vi "Broadcast Refnum.vi"(8 "error in":errorcluster) -> (0 "error out":errorcluster, 3 "Broadcast Refnum":T1)   [LabVIEW 2020, in "SECS Scenarios.lvlib" / "Scenarios Class.lvclass"]
uses:
  Scenarios Class.lvclass
  Broadcast Refnum.ctl
  13-EnableDisable Alarm.ctl
  15-Process Program Request.ctl
  16-Process Program Send.ctl
  SECS Communication/S7 Message Class/S7F4.ctl
  17-Deleting a Process Program by Host.ctl
  SECS Communication/S7 Message Class/S7F18.ctl
  18-Host Requests Equipment Process Program Directory.ctl
  19-Equipment Process Program Uploading.ctl
  SECS Communication/SECS-II Class/Format Code.ctl
  20[1]-Process Program Downloading.ctl
  SECS Communication/S7 Message Class/S7F2.ctl
  20[2]-Process Program Downloading.ctl
  SECS Communication/S7 Message Class/S7F23.ctl
  SECS Communication/S7 Message Class/S7F24.ctl
  22-Host Sends Information to Equipment.ctl
  SECS Communication/S10 Message Class/S10F4.ctl
  26-Host Requests to Enter OFF-Line.ctl
  27-Host Requests to Enter On-Line.ctl
  SECS Communication/S1 Message Class/S1F18.ctl
  28[1]-Remote Control[PP-SELECT].ctl
  28[2]-Remote Control[START].ctl
  28[3]-Remote Control[STOP].ctl
  28[4]-Remote Control[LOCAL].ctl
  28[5]-Remote Control[REMOTE].ctl
  28[6]-Remote Control[RCMD].ctl
  SECS Communication/S2 Message Class/S2F41.ctl
  SECS Communication/S2 Message Class/S2F42.ctl
  30-Host Requests Equipment to Set Time.ctl
  SECS Communication/S2 Message Class/S2F32.ctl
  31-Host Requests Time Value from Equipment.ctl
  32[1]-Trace Data Collection.ctl
  32[2]-Trace Data Collection.ctl
  SECS Communication/S2 Message Class/S2F24.ctl
  SECS Communication/S7 Message Class/S7 Message Class.lvclass
  SECS Communication/SECS-II Class/SECS-II Class.lvclass
  SECS Communication/S10 Message Class/S10 Message Class.lvclass
  SECS Communication/S1 Message Class/S1 Message Class.lvclass
  <vilib>/Utility/Data Type/NI_Data Type.lvlib
  SECS Communication/S2 Message Class/S2 Message Class.lvclass
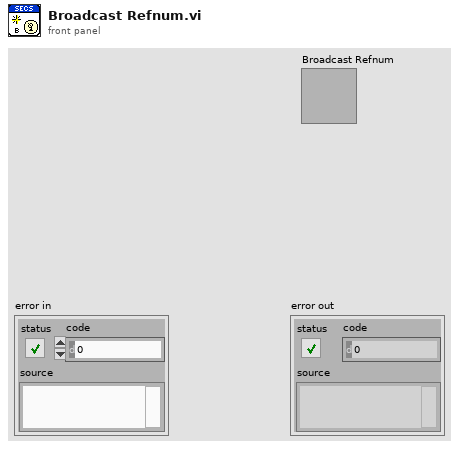
[diagram p1: front panel]
types:
  T1 = typedef "SECS Scenarios.lvlib/Scenarios Class.lvclass/Broadcast Refnum.ctl" = cluster{"13-EnableDisable Alarm":refnum<user-event>, "15-Process Program Request":refnum<user-event>, "16-Process Program Send":refnum<user-event>, "17-Deleting a Process Program by Host":refnum<user-event>, "18-Host Requests Equipment Process Program Directory":refnum<user-event>, "19-Equipment Process Program Uploading":refnum<user-event>, "20[1]-Process Program Downloading":refnum<user-event>, "20[2]-Process Program Downloading":refnum<user-event>, "22-Host Sends Information to Equipment":refnum<user-event>, "26-Host Requests to Enter OFF-Line":refnum<user-event>, "27-Host Requests to Enter On-Line":refnum<user-event>, "28[1]-Remote Control[PP-SELECT]":refnum<user-event>, "28[2]-Remote Control[START]":refnum<user-event>, "28[3]-Remote Control[STOP]":refnum<user-event>, "28[4]-Remote Control[LOCAL]":refnum<user-event>, "28[5]-Remote Control[REMOTE]":refnum<user-event>, "28[6]-Remote Control[RCMD]":refnum<user-event>, "30-Host Requests Equipment to Set Time":refnum<user-event>, "31-Host Requests Time Value from Equipment":refnum<user-event>, "32[1]-Trace Data Collection":refnum<user-event>, "32[2]-Trace Data Collection":refnum<user-event>}
  T2 = typedef "SECS Scenarios.lvlib/Scenarios Class.lvclass/13-EnableDisable Alarm.ctl" = cluster{"ALED":bool, "ALID":u32, "Reply Notifier":refnum<notifier>}
  T3 = typedef "SECS Scenarios.lvlib/Scenarios Class.lvclass/15-Process Program Request.ctl" = cluster{"PPID":string, "Reply Notifier":refnum<notifier>}
  T4 = typedef "SECS Scenarios.lvlib/Scenarios Class.lvclass/16-Process Program Send.ctl" = cluster{"PPID":string, "PPBODY":u8[], "Reply Notifier":refnum<notifier>}
  T5 = typedef "SECS Scenarios.lvlib/Scenarios Class.lvclass/17-Deleting a Process Program by Host.ctl" = cluster{"PPID":string[], "Reply Notifier":refnum<notifier>}
  T6 = typedef "SECS Scenarios.lvlib/Scenarios Class.lvclass/18-Host Requests Equipment Process Program Directory.ctl" = cluster{"Reply Notifier":refnum<notifier>}
  T7 = typedef "SECS Scenarios.lvlib/Scenarios Class.lvclass/19-Equipment Process Program Uploading.ctl" = cluster{"PPID":string, "Reply Notifier":refnum<notifier>}
  T8 = typedef "SECS Scenarios.lvlib/Scenarios Class.lvclass/20[1]-Process Program Downloading.ctl" = cluster{"PPID":string, "LENGTH":u32, "Reply Notifier":refnum<notifier>}
  T9 = typedef "SECS Scenarios.lvlib/Scenarios Class.lvclass/20[2]-Process Program Downloading.ctl" = cluster{"S7F23":T10, "Reply Notifier":refnum<notifier>}
  T10 = typedef "SECS Communication.lvlib/S7 Message Class.lvclass/S7F23.ctl" = cluster{"PPID":string, "MDLN":string, "SOFTREV":string, "Parameter":cluster{"CCODE":string, "PPARM":cluster{"Format Code":T11, "Value":variant}[]}[]}
  T11 = typedef "SECS Communication.lvlib/SECS-II Class.lvclass/Format Code.ctl" = enum16{"L", "A", "B", "Boolean", "J", "I1", "I2", "I4", "I8", "U1", "U2", "U4", "U8", "F4", "F8", "Char"}
  T12 = typedef "SECS Scenarios.lvlib/Scenarios Class.lvclass/22-Host Sends Information to Equipment.ctl" = cluster{"TID":u8, "TEXT":string, "Reply Notifier":refnum<notifier>}
  T13 = typedef "SECS Scenarios.lvlib/Scenarios Class.lvclass/26-Host Requests to Enter OFF-Line.ctl" = cluster{"Off-Line":bool, "Reply Notifier":refnum<notifier>}
  T14 = typedef "SECS Scenarios.lvlib/Scenarios Class.lvclass/27-Host Requests to Enter On-Line.ctl" = cluster{"On-Line":bool, "Reply Notifier":refnum<notifier>}
  T15 = typedef "SECS Scenarios.lvlib/Scenarios Class.lvclass/28[1]-Remote Control[PP-SELECT].ctl" = cluster{"PPID":string, "Reply Notifier":refnum<notifier>}
  T16 = typedef "SECS Scenarios.lvlib/Scenarios Class.lvclass/28[2]-Remote Control[START].ctl" = cluster{"Reply Notifier":refnum<notifier>}
  T17 = typedef "SECS Scenarios.lvlib/Scenarios Class.lvclass/28[3]-Remote Control[STOP].ctl" = cluster{"Reply Notifier":refnum<notifier>}
  T18 = typedef "SECS Scenarios.lvlib/Scenarios Class.lvclass/28[4]-Remote Control[LOCAL].ctl" = cluster{"Reply Notifier":refnum<notifier>}
  T19 = typedef "SECS Scenarios.lvlib/Scenarios Class.lvclass/28[5]-Remote Control[REMOTE].ctl" = cluster{"Reply Notifier":refnum<notifier>}
  T20 = typedef "SECS Scenarios.lvlib/Scenarios Class.lvclass/28[6]-Remote Control[RCMD].ctl" = cluster{"S2F41":T21, "Reply Notifier":refnum<notifier>}
  T21 = typedef "SECS Communication.lvlib/S2 Message Class.lvclass/S2F41.ctl" = cluster{"RCMD":string, "Parameter":cluster{"CPNAME":string, "CPVAL":string}[]}
  T22 = typedef "SECS Scenarios.lvlib/Scenarios Class.lvclass/30-Host Requests Equipment to Set Time.ctl" = cluster{"Time":string, "Reply Notifier":refnum<notifier>}
  T23 = typedef "SECS Scenarios.lvlib/Scenarios Class.lvclass/31-Host Requests Time Value from Equipment.ctl" = cluster{"Reply Notifier":refnum<notifier>}
  T24 = typedef "SECS Scenarios.lvlib/Scenarios Class.lvclass/32[1]-Trace Data Collection.ctl" = cluster{"Terminate TRID":u32}
  T25 = typedef "SECS Scenarios.lvlib/Scenarios Class.lvclass/32[2]-Trace Data Collection.ctl" = cluster{"TRID":u32, "DSPER":string, "TOTSMP":u32, "REPGSZ":u32, "SVID":u32[], "Reply Notifier":refnum<notifier>}
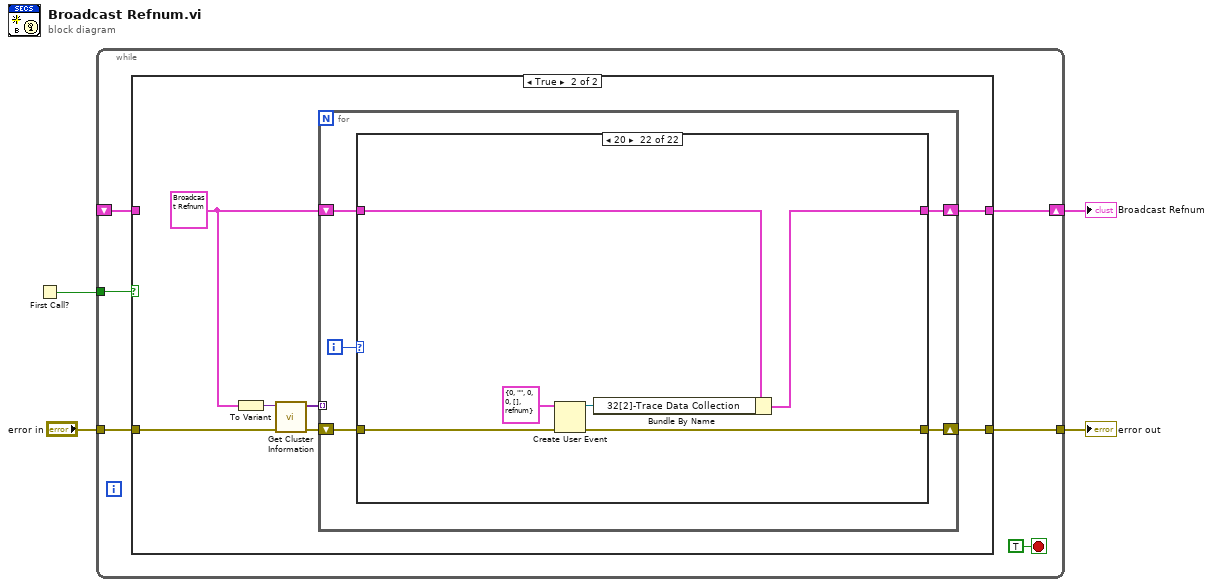
[diagram p0: block diagram]
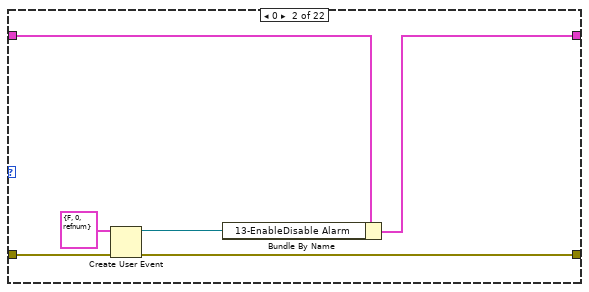
[diagram p4: hidden frame]
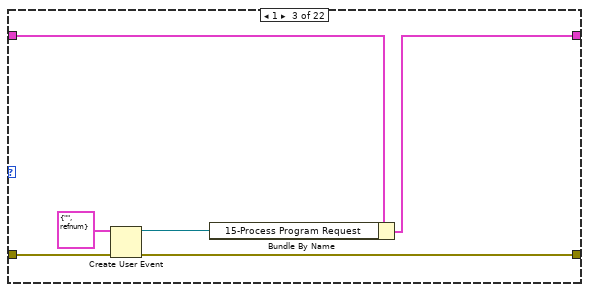
[diagram p5: hidden frame]
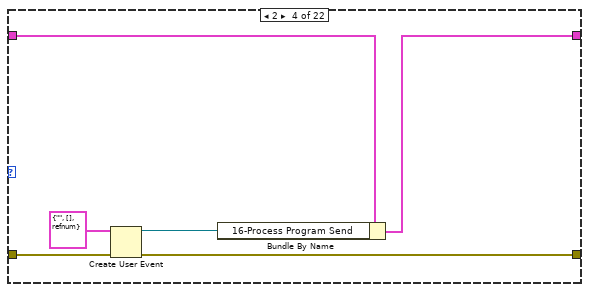
[diagram p6: hidden frame]
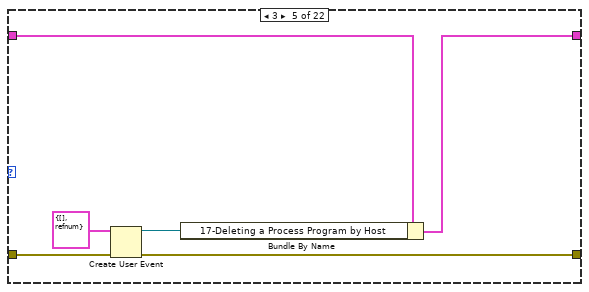
[diagram p7: hidden frame]
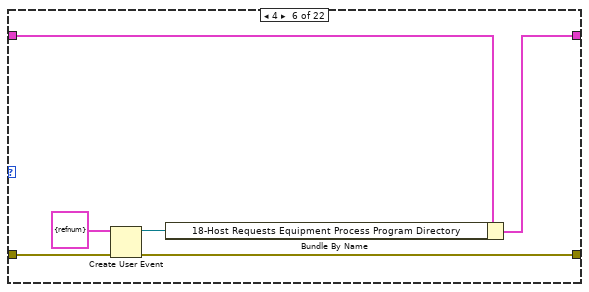
[diagram p8: hidden frame]
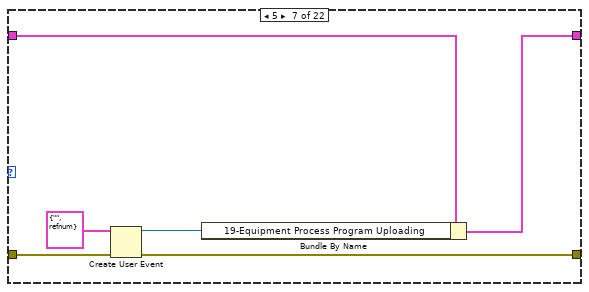
[diagram p9: hidden frame]
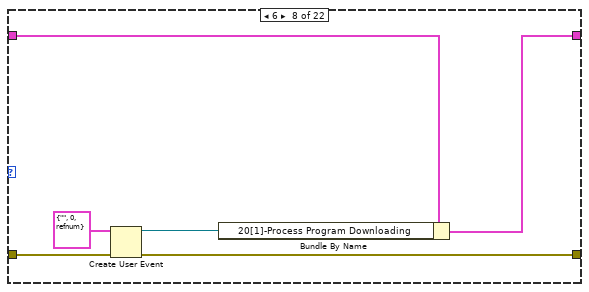
[diagram p10: hidden frame]
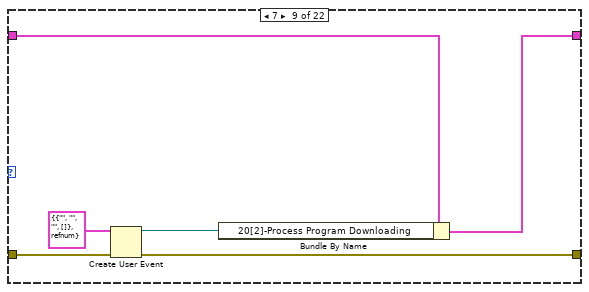
[diagram p11: hidden frame]
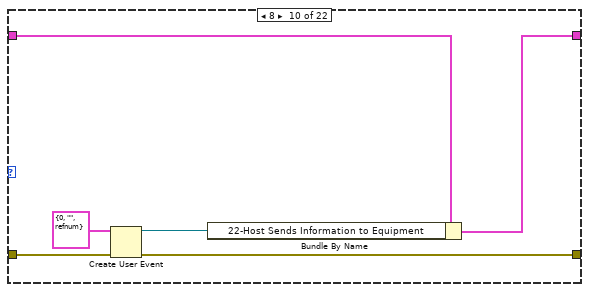
[diagram p12: hidden frame]
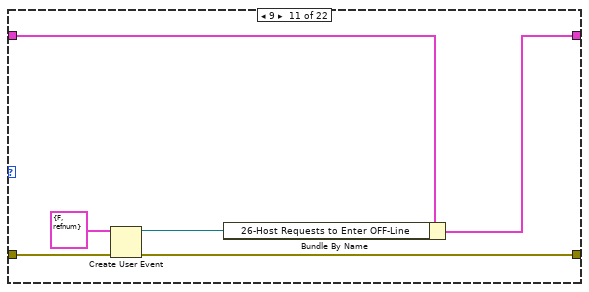
[diagram p13: hidden frame]
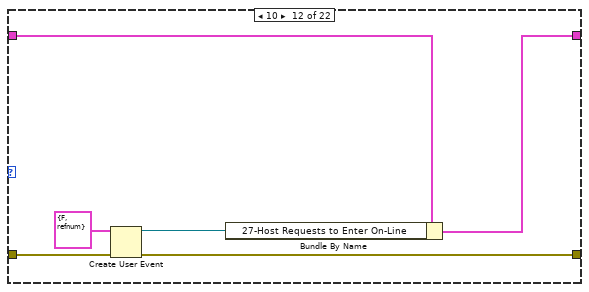
[diagram p14: hidden frame]
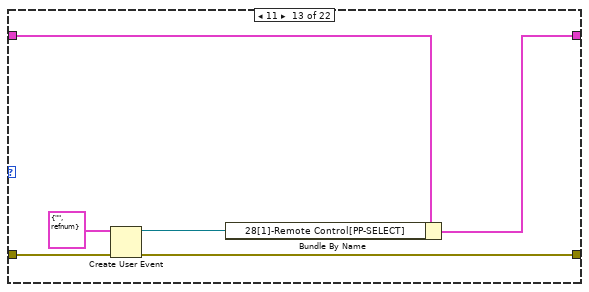
[diagram p15: hidden frame]
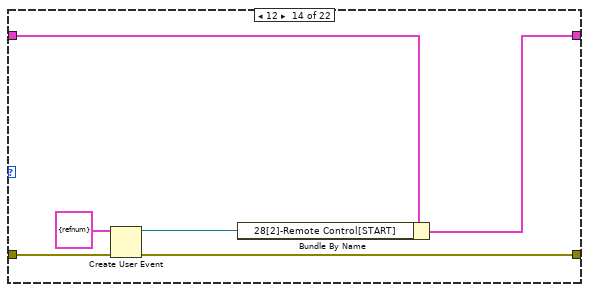
[diagram p16: hidden frame]
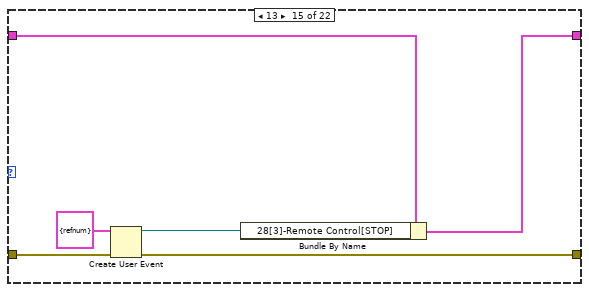
[diagram p17: hidden frame]
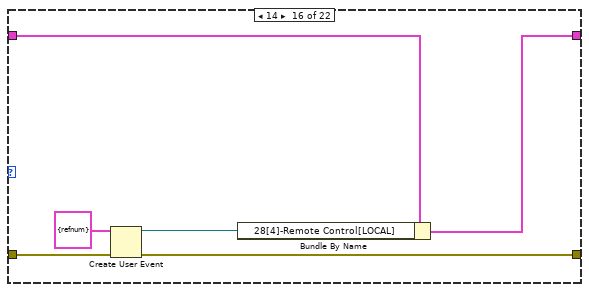
[diagram p18: hidden frame]
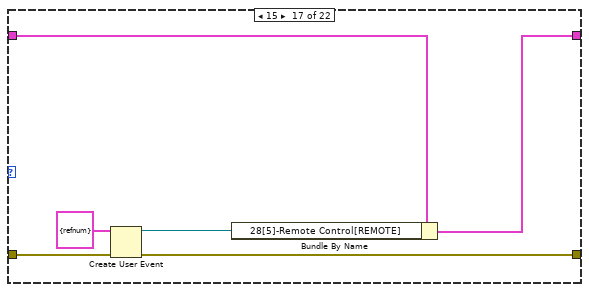
[diagram p19: hidden frame]
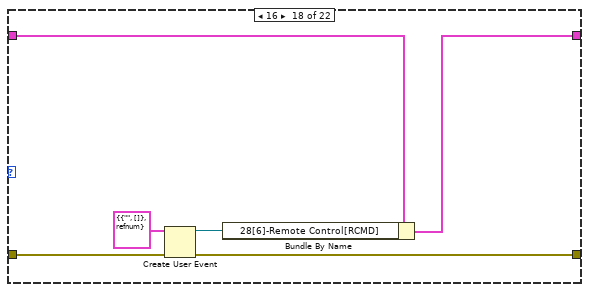
[diagram p20: hidden frame]
diagram:
  n1 = First Call?() -> (First Call?: T/F=w3:bool)
  n2 = while {
    tunnel: "error in" -> [w9]
    tunnel: w3 -> [w10]
    tunnel: [w8] -> w2
    shift-right: [w7] -> w1
    shift-left: _ -> [w6]
    stop <- TRUE stop-if-true
    n3 = case shown="True" w10 {
      tunnel: w9 -> [w11 w19]
      tunnel: [w11 w13] -> w8
      tunnel: [w12 w14] -> w7
      tunnel: w6 -> [w12 _]
      frame False {
      }
      frame True {
        w15 = T1 {"13-EnableDisable Alarm"=refnum, "15-Process Program Request"=refnum, "16-Process Program Send"=refnum, "17-Deleting a Process Program by Host"=refnum, "18-Host Requests Equipment Process Program Directory"=refnum, "19-Equipment Process Program Uploading"=refnum, "20[1]-Process Program Downloading"=refnum, "20[2]-Process Program Downloading"=refnum, "22-Host Sends Information to Equipment"=refnum, "26-Host Requests to Enter OFF-Line"=refnum, "27-Host Requests to Enter On-Line"=refnum, "28[1]-Remote Control[PP-SELECT]"=refnum, "28[2]-Remote Control[START]"=refnum, "28[3]-Remote Control[STOP]"=refnum, "28[4]-Remote Control[LOCAL]"=refnum, "28[5]-Remote Control[REMOTE]"=refnum, "28[6]-Remote Control[RCMD]"=refnum, "30-Host Requests Equipment to Set Time"=refnum, "31-Host Requests Time Value from Equipment"=refnum, "32[1]-Trace Data Collection"=refnum, "32[2]-Trace Data Collection"=refnum} ("User Event Refnum")
        n4 = To Variant(anything=w15) -> (Variant=w18:variant)
        n5 = call <vilib>:"Get Cluster Information.vi"("error in (no error)"=w19, "variant"=w18) -> ("error out"=w17:errorcluster, "cluster elements"=w16:variant[])  [unwired: 8 in]
        n6 = for {
          tunnel: w16 -> [_] mode=indexing
          shift-right: [w21] -> w14
          shift-left: w15 -> [w23]
          shift-right: [w20] -> w13
          shift-left: w17 -> [w24]
          i -> [w22]
          n7 = case shown="20" w22 {
            tunnel: w24 -> [w25 w31 w38 w44 w50 w56 w62 w68 w74 w80 w86 w92 w98 w104 w110 w116 w122 w125 w134 w140 w146 w152]
            tunnel: w23 -> [w26 w30 w37 w43 w49 w55 w61 w67 w73 w79 w85 w91 w97 w103 w109 w115 w121 w128 w133 w139 w145 w151]
            tunnel: [w26 w27 w34 w40 w46 w52 w58 w64 w70 w76 w82 w88 w94 w100 w107 w113 w119 w127 w131 w137 w143 w149] -> w21
            tunnel: [w25 w28 w35 w41 w47 w53 w59 w65 w71 w77 w83 w89 w95 w101 w108 w114 w120 w124 w132 w138 w144 w150] -> w20
            frame Default {
            }
            frame 0 {
              n8 = Create User Event(user event datatype=T2 {"ALED"=FALSE, "ALID"=0, "Reply Notifier"=refnum} ("13-EnableDisable Alarm"), error in=w31) -> (user event=w29:refnum<user-event>, error out=w28:errorcluster)
              n9 = Bundle By Name(cluster=w30, "13-EnableDisable Alarm"=w29) -> (w27:T1)
            }
            frame 1 {
              n10 = Create User Event(user event datatype=T3 {"PPID"="", "Reply Notifier"=refnum} ("15-Process Program Request"), error in=w38) -> (user event=w36:refnum<user-event>, error out=w35:errorcluster)
              n11 = Bundle By Name(cluster=w37, "15-Process Program Request"=w36) -> (w34:T1)
            }
            frame 2 {
              n12 = Create User Event(user event datatype=T4 {"PPID"="", "PPBODY"=[], "Reply Notifier"=refnum} ("16-Process Program Send"), error in=w44) -> (user event=w42:refnum<user-event>, error out=w41:errorcluster)
              n13 = Bundle By Name(cluster=w43, "16-Process Program Send"=w42) -> (w40:T1)
            }
            frame 3 {
              n14 = Create User Event(user event datatype=T5 {"PPID"=[], "Reply Notifier"=refnum} ("17-Deleting a Process Program by Host"), error in=w50) -> (user event=w48:refnum<user-event>, error out=w47:errorcluster)
              n15 = Bundle By Name(cluster=w49, "17-Deleting a Process Program by Host"=w48) -> (w46:T1)
            }
            frame 4 {
              n16 = Create User Event(user event datatype=T6 {"Reply Notifier"=refnum} ("18-Host Requests Equipment Process Program Directory"), error in=w56) -> (user event=w54:refnum<user-event>, error out=w53:errorcluster)
              n17 = Bundle By Name(cluster=w55, "18-Host Requests Equipment Process Program Directory"=w54) -> (w52:T1)
            }
            frame 5 {
              n18 = Create User Event(user event datatype=T7 {"PPID"="", "Reply Notifier"=refnum} ("19-Equipment Process Program Uploading"), error in=w62) -> (user event=w60:refnum<user-event>, error out=w59:errorcluster)
              n19 = Bundle By Name(cluster=w61, "19-Equipment Process Program Uploading"=w60) -> (w58:T1)
            }
            frame 6 {
              n20 = Create User Event(user event datatype=T8 {"PPID"="", "LENGTH"=0, "Reply Notifier"=refnum} ("20[1]-Process Program Downloading"), error in=w68) -> (user event=w66:refnum<user-event>, error out=w65:errorcluster)
              n21 = Bundle By Name(cluster=w67, "20[1]-Process Program Downloading"=w66) -> (w64:T1)
            }
            frame 7 {
              n22 = Create User Event(user event datatype=T9 {"S7F23"={"PPID"="", "MDLN"="", "SOFTREV"="", "Parameter"=[]}, "Reply Notifier"=refnum} ("20[2]-Process Program Downloading"), error in=w74) -> (user event=w72:refnum<user-event>, error out=w71:errorcluster)
              n23 = Bundle By Name(cluster=w73, "20[2]-Process Program Downloading"=w72) -> (w70:T1)
            }
            frame 8 {
              n24 = Create User Event(user event datatype=T12 {"TID"=0, "TEXT"="", "Reply Notifier"=refnum} ("22-Host Sends Information to Equipment"), error in=w80) -> (user event=w78:refnum<user-event>, error out=w77:errorcluster)
              n25 = Bundle By Name(cluster=w79, "22-Host Sends Information to Equipment"=w78) -> (w76:T1)
            }
            frame 9 {
              n26 = Create User Event(user event datatype=T13 {"Off-Line"=FALSE, "Reply Notifier"=refnum} ("26-Host Requests to Enter OFF-Line"), error in=w86) -> (user event=w84:refnum<user-event>, error out=w83:errorcluster)
              n27 = Bundle By Name(cluster=w85, "26-Host Requests to Enter OFF-Line"=w84) -> (w82:T1)
            }
            frame 10 {
              n28 = Create User Event(user event datatype=T14 {"On-Line"=FALSE, "Reply Notifier"=refnum} ("27-Host Requests to Enter On-Line"), error in=w92) -> (user event=w90:refnum<user-event>, error out=w89:errorcluster)
              n29 = Bundle By Name(cluster=w91, "27-Host Requests to Enter On-Line"=w90) -> (w88:T1)
            }
            frame 11 {
              n30 = Create User Event(user event datatype=T15 {"PPID"="", "Reply Notifier"=refnum} ("28[1]-Remote Control[PP-SELECT]"), error in=w98) -> (user event=w96:refnum<user-event>, error out=w95:errorcluster)
              n31 = Bundle By Name(cluster=w97, "28[1]-Remote Control[PP-SELECT]"=w96) -> (w94:T1)
            }
            frame 12 {
              n32 = Create User Event(user event datatype=T16 {"Reply Notifier"=refnum} ("28[2]-Remote Control[START]"), error in=w104) -> (user event=w102:refnum<user-event>, error out=w101:errorcluster)
              n33 = Bundle By Name(cluster=w103, "28[2]-Remote Control[START]"=w102) -> (w100:T1)
            }
            frame 13 {
              n34 = Create User Event(user event datatype=T17 {"Reply Notifier"=refnum} ("28[3]-Remote Control[STOP]"), error in=w110) -> (user event=w105:refnum<user-event>, error out=w108:errorcluster)
              n35 = Bundle By Name(cluster=w109, "28[3]-Remote Control[STOP]"=w105) -> (w107:T1)
            }
            frame 14 {
              n36 = Create User Event(user event datatype=T18 {"Reply Notifier"=refnum} ("28[4]-Remote Control[LOCAL]"), error in=w116) -> (user event=w111:refnum<user-event>, error out=w114:errorcluster)
              n37 = Bundle By Name(cluster=w115, "28[4]-Remote Control[LOCAL]"=w111) -> (w113:T1)
            }
            frame 15 {
              n38 = Create User Event(user event datatype=T19 {"Reply Notifier"=refnum} ("28[5]-Remote Control[REMOTE]"), error in=w122) -> (user event=w117:refnum<user-event>, error out=w120:errorcluster)
              n39 = Bundle By Name(cluster=w121, "28[5]-Remote Control[REMOTE]"=w117) -> (w119:T1)
            }
            frame 16 {
              n40 = Create User Event(user event datatype=T20 {"S2F41"={"RCMD"="", "Parameter"=[]}, "Reply Notifier"=refnum} ("28[6]-Remote Control[RCMD]"), error in=w125) -> (user event=w123:refnum<user-event>, error out=w124:errorcluster)
              n41 = Bundle By Name(cluster=w128, "28[6]-Remote Control[RCMD]"=w123) -> (w127:T1)
            }
            frame 17 {
              n42 = Create User Event(user event datatype=T22 {"Time"="", "Reply Notifier"=refnum} ("30-Host Requests Equipment to Set Time"), error in=w134) -> (user event=w130:refnum<user-event>, error out=w132:errorcluster)
              n43 = Bundle By Name(cluster=w133, "30-Host Requests Equipment to Set Time"=w130) -> (w131:T1)
            }
            frame 18 {
              n44 = Create User Event(user event datatype=T23 {"Reply Notifier"=refnum} ("31-Host Requests Time Value from Equipment"), error in=w140) -> (user event=w136:refnum<user-event>, error out=w138:errorcluster)
              n45 = Bundle By Name(cluster=w139, "31-Host Requests Time Value from Equipment"=w136) -> (w137:T1)
            }
            frame 19 {
              n46 = Create User Event(user event datatype=T24 {"Terminate TRID"=1} ("32[1]-Trace Data Collection"), error in=w146) -> (user event=w141:refnum<user-event>, error out=w144:errorcluster)
              n47 = Bundle By Name(cluster=w145, "32[1]-Trace Data Collection"=w141) -> (w143:T1)
            }
            frame 20 {
              n48 = Create User Event(user event datatype=T25 {"TRID"=0, "DSPER"="", "TOTSMP"=0, "REPGSZ"=0, "SVID"=[], "Reply Notifier"=refnum} ("32[2]-Trace Data Collection"), error in=w152) -> (user event=w147:refnum<user-event>, error out=w150:errorcluster)
              n49 = Bundle By Name(cluster=w151, "32[2]-Trace Data Collection"=w147) -> (w149:T1)
            }
          }
        }
      }
    }
  }
  "error out" <- w2
  "Broadcast Refnum" <- w1
